vi "TBControlCheck_ver1.0.vi"(0 "output cluster":T1={"Main Sweep"=0, "Steps Config:"={"total points:"=0, "Step Delay (s)"=0.0, "Ini Delay (s)"=0.0, "# of steps:"=0}, "Temperature Control (ITC 503):"={"GPIB ADR"=0, "Change Heater?"={"Heater?"=FALSE, "Heater"=0}, "Change Temp?"={"Change T?"=FALSE, "Set T (K)"=0.0}, "Cluster"={"Heat Auto?"=FALSE, "Manual Heat?"=FALSE, "Heater (%)"=0.0}, "Change PID?"={"Change PID?"=FALSE, "P"=0.0, "I"=0.0, "D"=0.0}, "Change Para?"=FALSE, "Sensor"=1}, "Temperature Control (LS 340):"={"GPIB ADR"=0, "From (K)"=0.0, "To (K)"=0.0, "Rate (K/min)"=0.0, "Delta T (0.08K)"=0.0, "Temp. Header"="", "T Display Control"={"Ch B"=FALSE, "Ch C"=FALSE, "Ch D"=FALSE}}, "Magnet Control (IPS 120-10)"={"Action"=0, "Standby (s)"=0.0, "Heater on (s)"=0.0, "Sweep Setup "=[], "GPIB ADR"=0, "Change Para?"=FALSE}, "Keithley 6221 :"=[], "Measuring Instruments : "=[], "Lock-In SR7265 :"=[], "Deascription of \nthis measurement"="", "Instruments Config:"=[], "LS372 Bridge : 2"=[{"GPIB"=0, "Excitation"=0, "Autorange?"=FALSE, "Range"=0, "Current"=0, "Voltage"=0, "DataHeader"="Rx;Ry"}], "Magnet Control (CS4) 2"={"Action"=1, "Standby (s)"=0.0, "Heater on (s)"=300.0, "Sweep Setup "=[], "GPIB ADR"=0, "Change Para?"=FALSE}} {"Magnet Control (CS4) 2"."GPIB ADR" items=["None"=0, "25"=25]; "Magnet Control (CS4) 2"."Sweep Setup"."Rate in Range (T/min)" min=0.001 max=0.5 step=0.001; "Magnet Control (CS4) 2"."Sweep Setup"."Hold(min)" min=0.0; "Magnet Control (CS4) 2"."Sweep Setup"."Set Point (T)" min=-9.0 max=9.0 step=0.001; "Magnet Control (CS4) 2"."Action" items=["Up", "Down", "Pause", "Zero"]; "LS372 Bridge : 2"."Voltage" items=["2.00 uV"=1, "6.32 uV"=2, "20.0 uV"=3, "63.2 uV"=4, "200 uV"=5, "632 uV"=6, "2.0 mV"=7, "6.32 mV"=8]; "LS372 Bridge : 2"."Current" items=["1.00 pA"=1, "3.16 pA"=2, "10.0 pA"=3, "31.6 pA"=4, "100 pA"=5, "316 pA"=6, "1.00 nA"=7, "3.16 nA"=8, "10 nA"=9, "31.6 nA"=10, "100 nA"=11, "316 nA"=12, "1.00 uA"=13, "3.16 uA"=14, "10.0 uA"=15, "31.6 uA"=16, "100 uA"=17, "316 uA"=18, "1.00 mA"=19, "3.16 mA"=20, "10.0 mA"=21, "31.6 mA"=22]; "LS372 Bridge : 2"."Range" items=["2.0 m"=1, "6.32 m"=2, "20.0 m"=3, "63.2 m"=4, "200 m"=5, "632 m"=6, "2.00"=7, "6.32"=8, "20.0"=9, "63.2"=10, "200"=11, "632"=12, "2.00 k"=13, "6.32 k"=14, "20.0 k"=15, "63.2 k"=16, "200 k"=17, "632 k"=18, "2.00 M"=19, "6.32 M"=20, "20.0 M"=21, "63.2 M"=22]; "LS372 Bridge : 2"."Excitation" items=["Voltage", "Current"]; "LS372 Bridge : 2"."GPIB" items=["None"=0, "9"=9]; "Main Sweep" items=["Time", "DC Current", "Delta Current", "Pulse Delta Current", "Sine Current", "Lock-in Vosc"]; "Temperature Control (ITC 503):"."Sensor" items=["T2", "T3"]; "Magnet Control (IPS 120-10)"."Action" items=["Hold", "To Set point", "To Zero", "Clamp"]; "Keithley 6221 :"."Sweep Mode" items=["Linear", "Log", "Exp", "Inverse", "Manual"]}) -> (1 "T&B Setting Change?":bool, 2 "ITC503 Change Para?":bool, 3 "LS340 Change Para?":bool, 4 "IPS120 Change Para?":bool)   [LabVIEW 2012]
panel:
  out "CS4 Change Para?":bool
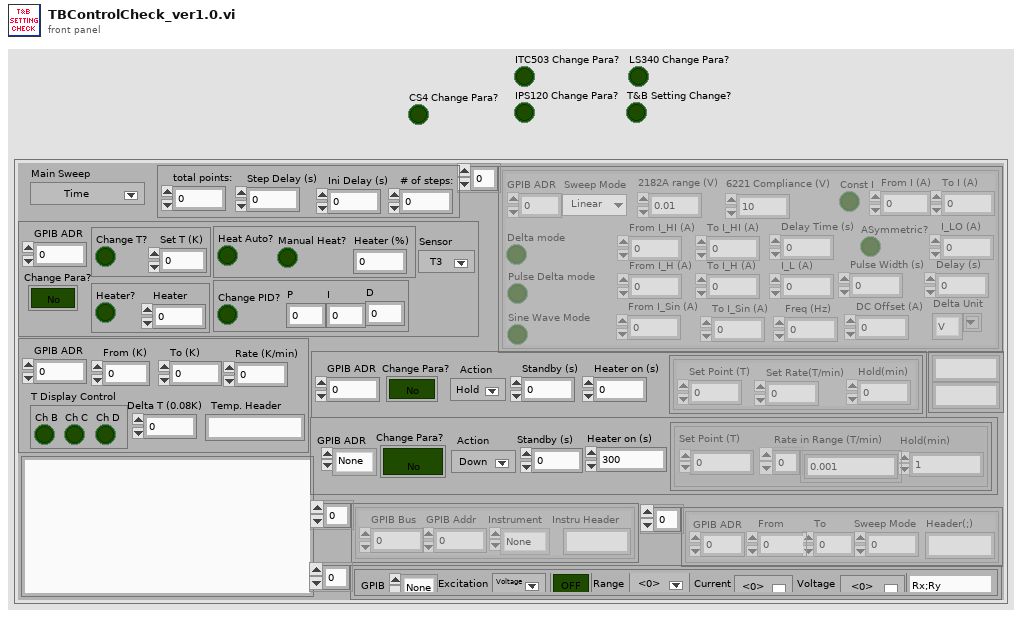
[diagram p1: front panel]
types:
  T1 = cluster{"Main Sweep":u8, "Steps Config:":cluster{"total points:":u32, "Step Delay (s)":dbl, "Ini Delay (s)":dbl, "# of steps:":u32}, "Temperature Control (ITC 503):":cluster{"GPIB ADR":u16, "Change Heater?":cluster{"Heater?":bool, "Heater":u8}, "Change Temp?":cluster{"Change T?":bool, "Set T (K)":dbl}, "Cluster":cluster{"Heat Auto?":bool, "Manual Heat?":bool, "Heater (%)":dbl}, "Change PID?":cluster{"Change PID?":bool, "P":dbl, "I":dbl, "D":dbl}, "Change Para?":bool, "Sensor":u16}, "Temperature Control (LS 340):":cluster{"GPIB ADR":u16, "From (K)":dbl, "To (K)":dbl, "Rate (K/min)":dbl, "Delta T (0.08K)":dbl, "Temp. Header":string, "T Display Control":cluster{"Ch B":bool, "Ch C":bool, "Ch D":bool}}, "Magnet Control (IPS 120-10)":cluster{"Action":u16, "Standby (s)":dbl, "Heater on (s)":dbl, "Sweep Setup ":cluster{"Set Point (T)":dbl, "Set Rate(T/min)":dbl, "Hold(min)":dbl}[], "GPIB ADR":u16, "Change Para?":bool}, "Keithley 6221 :":cluster{"Delta mode":bool, "Const I":bool, "Pulse Delta mode":bool, "Sine Wave Mode":bool, "From I_HI (A)":dbl, "From I (A)":dbl, "I_LO (A)":dbl, "From I_H (A)":dbl, "I_L (A)":dbl, "Freq (Hz)":dbl, "From I_Sin (A)":dbl, "DC Offset (A)":dbl, "Delay Time (s)":dbl, "Pulse Width (s)":dbl, "Delay (s)":dbl, "To I (A)":dbl, "ASymmetric?":bool, "To I_HI (A)":dbl, "To I_H (A)":dbl, "To I_Sin (A)":dbl, "GPIB ADR":u16, "Sweep Mode":u8, "Delta Unit":string, "2182A range (V)":dbl, "6221 Compliance (V)":dbl}[], "Measuring Instruments : ":cluster{"GPIB Bus":dbl, "GPIB Addr":dbl, "Instrument":enum16{"None", "HP34401DMM", "Lockin 7265", "HP3456/7A", "HP3478A", "HP3325FG", "Keithley2182A"}, "Instru Header":string}[], "Lock-In SR7265 :":cluster{"GPIB ADR":u16, "From":dbl, "To":dbl, "Header(;)":string, "Sweep Mode":u8}[], "Deascription of \nthis measurement":string, "Instruments Config:":string[][], "LS372 Bridge : 2":cluster{"GPIB":u16, "Excitation":u16, "Autorange?":bool, "Range":u16, "Current":u16, "Voltage":u16, "DataHeader":string}[], "Magnet Control (CS4) 2":cluster{"Action":u16, "Standby (s)":dbl, "Heater on (s)":dbl, "Sweep Setup ":cluster{"Set Point (T)":dbl, "Hold(min)":dbl, "Rate in Range (T/min)":dbl[]}[], "GPIB ADR":u16, "Change Para?":bool}}
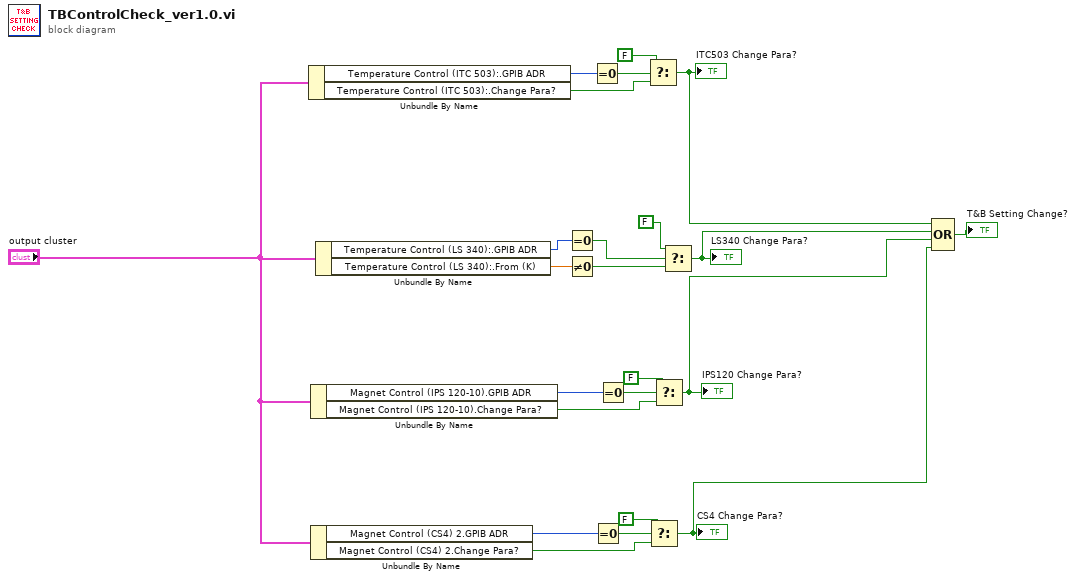
[diagram p0: block diagram]
diagram:
  n1 = Unbundle By Name("output cluster") -> ("Temperature Control (ITC 503):.GPIB ADR"=w23:u16, "Temperature Control (ITC 503):.Change Para?"=w20:bool)
  n2 = Unbundle By Name("output cluster") -> ("Magnet Control (IPS 120-10).GPIB ADR"=w22:u16, "Magnet Control (IPS 120-10).Change Para?"=w17:bool)
  n3 = Unbundle By Name("output cluster") -> ("Magnet Control (CS4) 2.GPIB ADR"=w3:u16, "Magnet Control (CS4) 2.Change Para?"=w2:bool)
  n4 = Unbundle By Name("output cluster") -> ("Temperature Control (LS 340):.GPIB ADR"=w14:u16, "Temperature Control (LS 340):.From (K)"=w15:dbl)
  n5 = Equal To 0?(x=w14) -> (x = 0?=w13:bool)
  n6 = Not Equal To 0?(x=w15) -> (x != 0?=w11:bool)
  n7 = Equal To 0?(x=w23) -> (x = 0?=w21:bool)
  n8 = Equal To 0?(x=w3) -> (x = 0?=w5:bool)
  n9 = Equal To 0?(x=w22) -> (x = 0?=w18:bool)
  n10 = Select(t=FALSE, s=w21, f=w20) -> (s? t:f=w10:bool)
  "ITC503 Change Para?" <- w10
  n11 = Select(t=FALSE, s=w5, f=w2) -> (s? t:f=w1:bool)
  "CS4 Change Para?" <- w1
  n12 = Select(t=FALSE, s=w18, f=w17) -> (s? t:f=w8:bool)
  "IPS120 Change Para?" <- w8
  n13 = Select(t=FALSE, s=w13, f=w11) -> (s? t:f=w9:bool)
  "LS340 Change Para?" <- w9
  n14 = Compound Arithmetic op=OR(w10, w9, w8, w1) -> (→"T&B Setting Change?":bool)
